vi "MA Scale Corrections.vi"(1 "RMC Calc Inputs":T1, 2 "Enable":bool=TRUE, 3 "MA Filter Size":i32=60, 8 "Reset":bool) -> (14 "RMC_Sm":dbl, 15 "RMC":dbl format="%.2f", 16 "Raw Weight":dbl format="%.2f", 17 "Corrected Weight":dbl format="%.2f", 18 "Wcomp":dbl, 19 "Wbouy":dbl)   [LabVIEW 2012]
uses:
  RMC Calc Inputs.ctl
  <vilib>/Analysis/baseanly.llb/Mean (DBL).vi
  <vilib>/Analysis/NI_AALBase.lvlib
panel:
  out "Smoothed Weight":dbl
  out "Count":dbl
  in  "Buoyancy Correction":T2={"Restriction"="3.75", "Bone Dry"=7.001999855041504, "Energie"=7, "Volume"=7.0, "IMC"=70.16566993034309, "Tamb"=70.16566993034309} {"Bone Dry" format="%.2f"}
  out "ColorW":bool
  in  "Period":u32
  in  "Data In":dbl[](array[numeric]) format="%.2f"
  out "Data Out":dbl[](array[numeric]) format="%.2f"
  in  "Compteur":u32
  in  "Bal_in":dbl=0.085 format="%.4f"
  out "Bal_out":dbl=0.085 format="%.4f"
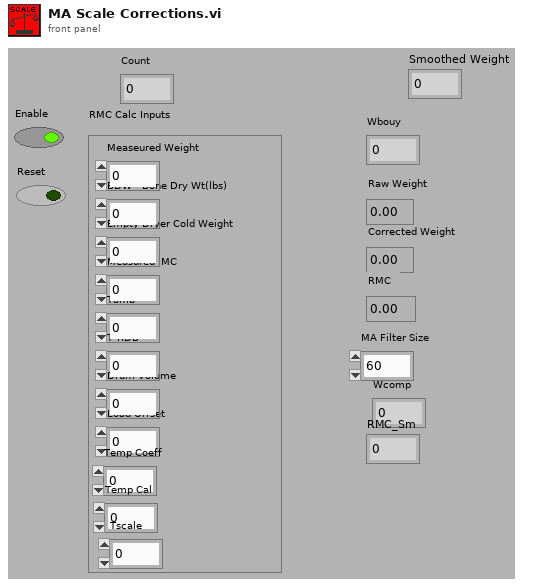
[diagram p1: front panel]
types:
  T1 = typedef "RMC Calc Inputs.ctl" = cluster{"Measeured Weight":dbl, "BDW - Bone Dry Wt(lbs)":dbl, "Empty Dryer Cold Weight":dbl, "Measured IMC":dbl, "Tamb":dbl, "T-RDB":dbl, "Drum Volume":dbl, "Load Offset":dbl, "Temp Coeff":dbl, "Temp Cal":dbl, "Tscale":dbl}
  T2 = cluster{"Restriction":string, "Bone Dry":dbl, "Energie":u8, "Volume":dbl, "IMC":dbl, "Tamb":dbl}
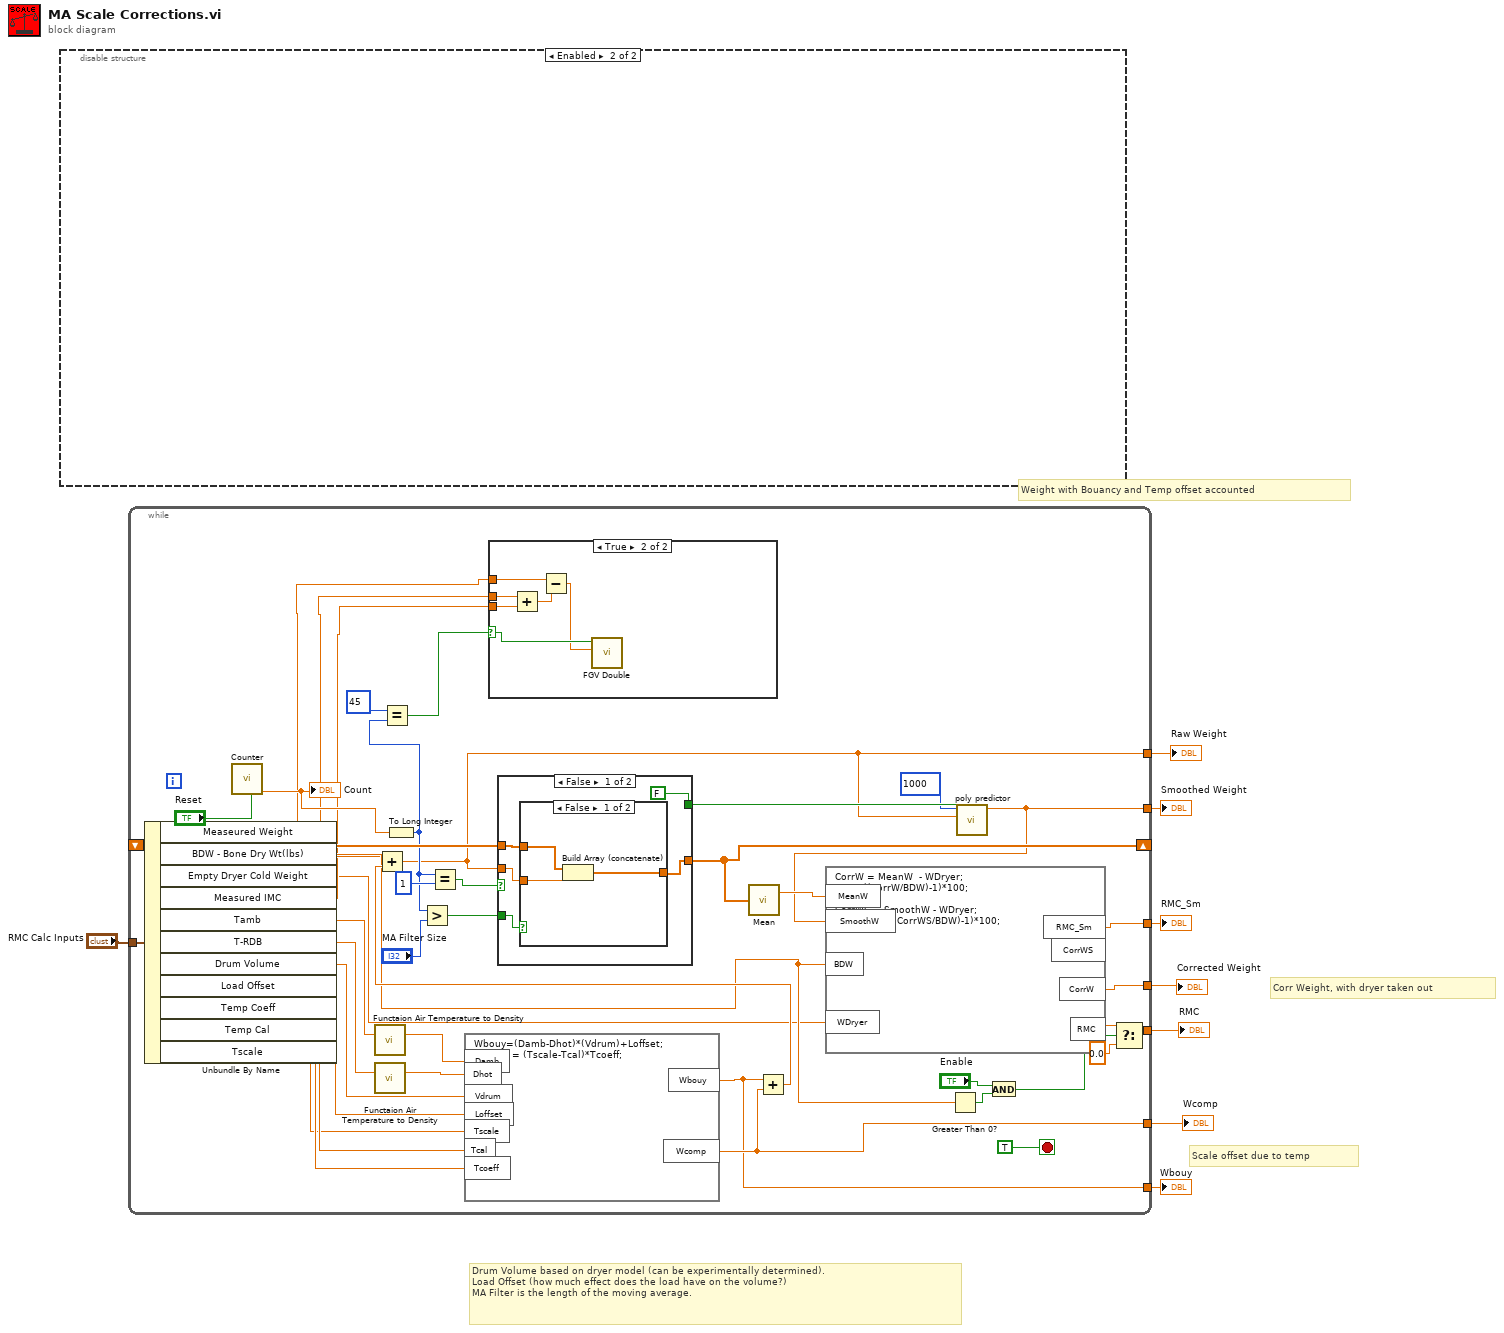
[diagram p0: block diagram]
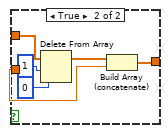
[diagram p3: hidden frame]
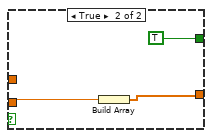
[diagram p4: hidden frame]
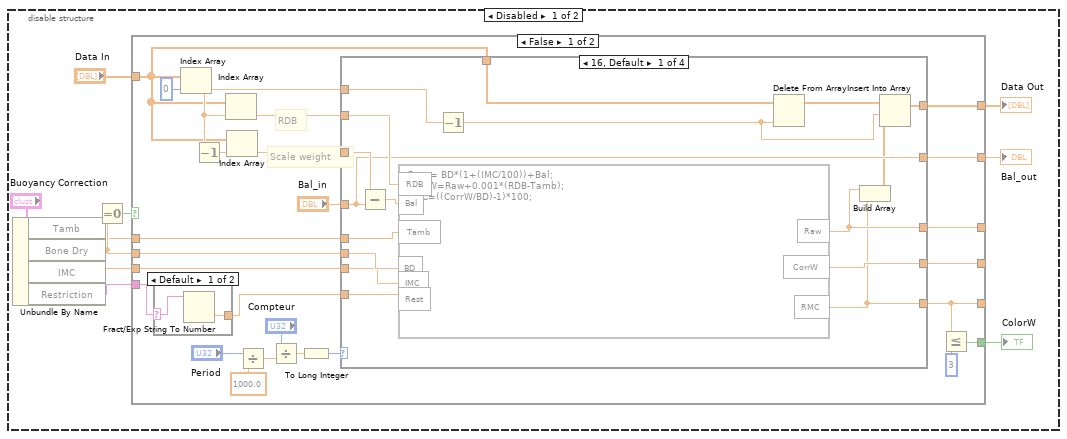
[diagram p5: hidden frame]
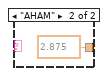
[diagram p6: hidden frame]
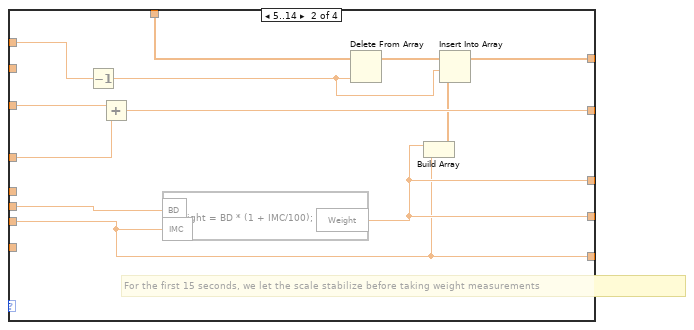
[diagram p7: hidden frame]
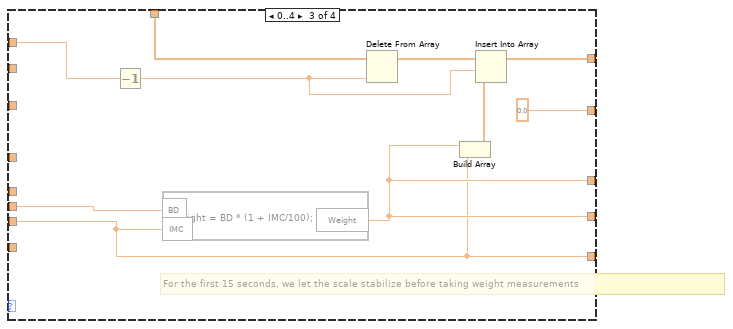
[diagram p8: hidden frame]
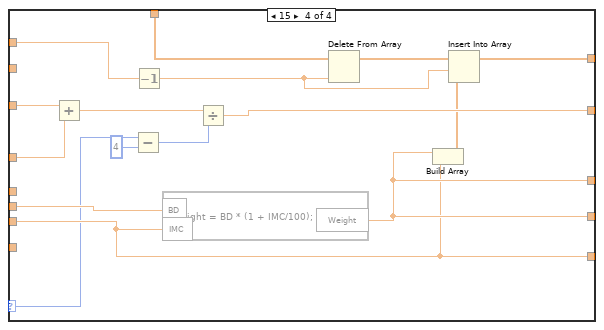
[diagram p9: hidden frame]
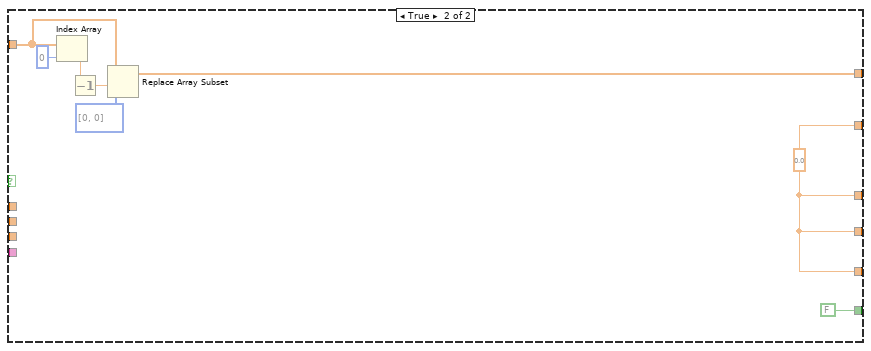
[diagram p10: hidden frame]
diagram:
  # "Corr Weight, with dryer taken out"
  # "Weight with Bouancy and Temp offset accounted"
  # "Scale offset due to temp"
  # "Drum Volume based on dryer model (can be experimentally determined).\nLoad Offset (how much effect does the load have on the volume?)\nMA Filter is the length of the moving average."
  n1 = disable-structure shown="Enabled" {
    frame Disabled {
      n2 = Unbundle By Name("Buoyancy Correction") -> ("Tamb"=w9:dbl, "Bone Dry"=w14:dbl, "IMC"=w13:dbl, "Restriction"=w12:string)
      n3 = Equal To 0?(x=w14) -> (x = 0?=w18:bool)
      n4 = case shown="False" w18 {
        tunnel: [w30 w103] -> _
        tunnel: [w29 w103] -> _
        tunnel: [w24 w103] -> _
        tunnel: "Data In" -> [w28 w107]
        tunnel: [w27 w104] -> w17
        tunnel: [w31 w103] -> w16
        tunnel: w14 -> [w26 _]
        tunnel: w13 -> [w25 _]
        tunnel: w12 -> [w21 _]
        tunnel: [w23 FALSE] -> w11
        tunnel: w9 -> [w19 _]
        frame False {
          # "RDB"
          # "Scale weight"
          n5 = case shown="Default" w21 {
            selector: w21 -> [w45 _]
            tunnel: [w44 2.875] -> w20
            frame Default {
              n6 = Fract/Exp String To Number(string=w45) -> (number=w44:dbl)  [unwired: 3 in, 1 out]
            }
            frame "AHAM" {
            }
          }
          n7 = Index Array(array=w28, index=0 ("Index")) -> (element=w41:dbl)
          n8 = Decrement(x=w41) -> (x-1=w42:dbl)
          n9 = Index Array(array=w28, index=w41) -> (element=w33:dbl)
          n10 = Index Array(array=w28, index=w42) -> (element=w34:dbl)
          n11 = Divide(x="Period", y=1000.0) -> (x/y=w38:dbl)
          n12 = Divide(x="Compteur", y=w38) -> (x/y=w36:dbl)
          n13 = To Long Integer(number=w36) -> (32bit integer=w37:i32)
          n14 = case shown="16, Default" w37 {
            selector: w37 -> [_ _ _ w89]
            tunnel: w34 -> [w58 w75 _ w101]
            tunnel: w33 -> [w60 _ _ _]
            tunnel: "Bal_in" -> [w57 w74 _ w100]
            tunnel: [w57 w73 0.0 ("Bal_in") w96] -> w31
            tunnel: w25 -> [w62 w66 w79 w91]
            tunnel: [w54 w66 w79 w91] -> w24
            tunnel: w26 -> [w63 w72 w85 w99]
            tunnel: w20 -> [w61 _ _ _]
            tunnel: [w55 w67 w80 w92] -> w30
            tunnel: [w56 w67 w80 w92] -> w29
            tunnel: w41 -> [w53 w69 w82 w95]
            tunnel: w28 -> [w52 w70 w83 w94]
            tunnel: [w50 w71 w84 w93] -> w27
            tunnel: w19 -> [w47 _ _ _]
            frame 16, Default {
              n15 = Subtract(x=w58, y=w57) -> (x-y=w59:dbl)
              n16 = formula code="Raw = BD*(1+(IMC/100))+Bal;\nCorrW=Raw+0.001*(RDB-Tamb);\nRMC=((CorrW/BD)-1)*100;"("Bal"=w59, "BD"=w63, "IMC"=w62, "Rest"=w61, "RDB"=w60, "Tamb"=w47) -> ("Raw"=w55:dbl, "CorrW"=w56:dbl, "RMC"=w54:dbl)
              n17 = Decrement(x=w53) -> (x-1=w48:dbl)
              n18 = Delete From Array(array=w52, index=w48) -> (array with subset deleted=w49:dbl[])  [unwired: 1 in, 1 out]
              n19 = Build Array(w55, w54) -> (w51:dbl[])
              n20 = Insert Into Array(array=w49, index=w48, new element=w51) -> (w50:dbl[])
            }
            frame 5..14 {
              # "For the first 15 seconds, we let the scale stabilize before taking weight measurements"
              n21 = Decrement(x=w69) -> (x-1=w64:dbl)
              n22 = Add(x=w75, y=w74) -> (x+y=w73:dbl)
              n23 = formula code="Weight = BD * (1 + IMC/100);"("BD"=w72, "IMC"=w66) -> ("Weight"=w67:dbl)
              n24 = Delete From Array(array=w70, index=w64) -> (array with subset deleted=w65:dbl[])  [unwired: 1 in, 1 out]
              n25 = Build Array(w67, w66) -> (w68:dbl[])
              n26 = Insert Into Array(array=w65, index=w64, new element=w68) -> (w71:dbl[])
            }
            frame 0..4 {
              # "For the first 15 seconds, we let the scale stabilize before taking weight measurements"
              n27 = Decrement(x=w82) -> (x-1=w76:dbl)
              n28 = formula code="Weight = BD * (1 + IMC/100);"("BD"=w85, "IMC"=w79) -> ("Weight"=w80:dbl)
              n29 = Delete From Array(array=w83, index=w76) -> (array with subset deleted=w77:dbl[])  [unwired: 1 in, 1 out]
              n30 = Build Array(w80, w79) -> (w81:dbl[])
              n31 = Insert Into Array(array=w77, index=w76, new element=w81) -> (w84:dbl[])
            }
            frame 15 {
              n32 = Add(x=w101, y=w100) -> (x+y=w98:dbl)
              n33 = Subtract(x=w89, y=4) -> (x-y=w97:i32)
              n34 = Decrement(x=w95) -> (x-1=w86:dbl)
              n35 = formula code="Weight = BD * (1 + IMC/100);"("BD"=w99, "IMC"=w91) -> ("Weight"=w92:dbl)
              n36 = Divide(x=w98, y=w97) -> (x/y=w96:dbl)
              n37 = Delete From Array(array=w94, index=w86) -> (array with subset deleted=w87:dbl[])  [unwired: 1 in, 1 out]
              n38 = Build Array(w92, w91) -> (w90:dbl[])
              n39 = Insert Into Array(array=w87, index=w86, new element=w90) -> (w93:dbl[])
            }
          }
          n40 = Less Or Equal?(x=w24, y=i8 3) -> (x <= y?=w23:bool)
        }
        frame True {
          w103 = 0.0
          n41 = Index Array(array=w107, index=0 ("Index")) -> (element=w108:dbl)
          n42 = Decrement(x=w108) -> (x-1=w106:dbl)
          n43 = Replace Array Subset(array=w107, new element=i32[] [0, 0] ("Array Constant"), index=w106) -> (w104:dbl[])
        }
      }
      "Data Out" <- w17
      "Bal_out" <- w16
      "ColorW" <- w11
    }
    frame Enabled {
    }
  }
  n44 = while {
    tunnel: "RMC Calc Inputs" -> [w150]
    shift-right: [w148] -> _
    shift-left: _ -> [w149]
    tunnel: [w130] -> w8
    tunnel: [w114] -> w7
    tunnel: [w146] -> w6
    tunnel: [w128] -> w4
    tunnel: [w122] -> w3
    tunnel: [w119] -> w2
    tunnel: [w117] -> w1
    stop <- TRUE stop-if-true
    n45 = Unbundle By Name(w150) -> ("Measeured Weight"=w112:dbl, "BDW - Bone Dry Wt(lbs)"=w124:dbl, "Empty Dryer Cold Weight"=w110:dbl, "Measured IMC"=w111:dbl, "Tamb"=w141:dbl, "T-RDB"=w140:dbl, "Drum Volume"=w138:dbl, "Load Offset"=w139:dbl, "Temp Coeff"=w135:dbl, "Temp Cal"=w134:dbl, "Tscale"=w132:dbl)
    n46 = call "Counter.vi"("Reset"="Reset") -> ("Count"=w123:dbl)  [unwired: 10 in]
    "Count" <- w123
    n47 = call "Functaion Air Temperature to Density.vi"("Temp(F)"=w141) -> ("Density (lb/ft3)"=w137:dbl)  [unwired: 14 in]
    n48 = call "Functaion Air Temperature to Density.vi"("Temp(F)"=w140) -> ("Density (lb/ft3)"=w136:dbl)  [unwired: 14 in]
    n49 = To Long Integer(number=w123) -> (32bit integer=w115:i32)
    n50 = Equal?(x=45 ("y"), y=w115) -> (x = y?=w113:bool)
    n51 = Greater?(x=w115, y="MA Filter Size") -> (0:w142:bool)
    n52 = Equal?(x=w115, y=1) -> (x = y?=w145:bool)
    n53 = formula code="Wbouy=(Damb-Dhot)*(Vdrum)+Loffset;\nWcomp = (Tscale-Tcal)*Tcoeff;"("Damb"=w137, "Dhot"=w136, "Vdrum"=w138, "Loffset"=w139, "Tscale"=w132, "Tcal"=w134, "Tcoeff"=w135) -> ("Wbouy"=w122:dbl, "Wcomp"=w128:dbl)
    n54 = case shown="True" w113 {
      selector: w113 -> [_ w157]
      tunnel: w112 -> [_ w156]
      tunnel: w111 -> [_ w155]
      tunnel: w110 -> [_ w154]
      frame False {
      }
      frame True {
        n55 = Add(x=w154, y=w155) -> (x+y=w153:dbl)
        n56 = Subtract(x=w156, y=w153) -> (x-y=w152:dbl)
        n57 = call "FGV Double.vi"("Value In"=w152, "Set?"=w157) -> ()  [unwired: 9 in, 1 out]
      }
    }
    n58 = Add(x=w122, y=w128) -> (x+y=w133:dbl)
    n59 = Add(x=w112, y=w133) -> (x+y=w114:dbl)
    n60 = case shown="False" w145 {
      tunnel: w114 -> [w162 w174]
      tunnel: w149 -> [w161 _]
      tunnel: [w160 w173] -> w148
      tunnel: w142 -> [w159 _]
      tunnel: [FALSE TRUE] -> w120
      frame False {
        n61 = case shown="False" w159 {
          tunnel: [w165 w166] -> w160
          tunnel: w162 -> [w164 w167]
          tunnel: w161 -> [w163 w171]
          frame False {
            n62 = Build Array (concatenate)(w163, w164) -> (w165:dbl[])
          }
          frame True {
            n63 = Delete From Array(array=w171, length=1, index=0) -> (array with subset deleted=w168:dbl[])  [unwired: 1 out]
            n64 = Build Array (concatenate)(w168, w167) -> (w166:dbl[])
          }
        }
      }
      frame True {
        n65 = Build Array(w174) -> (w173:dbl[])
      }
    }
    n66 = call-poly <vilib>:"Mean.vi"("X"=w148) -> ("mean"=w147:dbl)  [unwired: 1 out]
    n67 = Greater Than 0?(x=w124) -> (x > 0?=w126:bool)
    n68 = call "poly predictor.vi"("Initialize"=w120, "Weight"=w114, "Number of Values to Smooth"=1000) -> ("Smoothed Value"=w119:dbl)  [unwired: 8 in]
    n69 = formula code="CorrW = MeanW  - WDryer;\nRMC=((CorrW/BDW)-1)*100;\n\nCorrWS = SmoothW - WDryer;\nRMC_Sm = ((CorrWS/BDW)-1)*100;"("BDW"=w124, "MeanW"=w147, "WDryer"=w110, "SmoothW"=w119) -> ("CorrW"=w146:dbl, "RMC"=w131:dbl, "RMC_Sm"=w117:dbl)  [unwired: 1 out]
    n70 = And(x="Enable", y=w126) -> (x .and. y?=w125:bool)
    n71 = Select(t=w131, s=w125, f=0.0) -> (s? t:f=w130:dbl)
  }
  "RMC" <- w8
  "Corrected Weight" <- w6
  "Raw Weight" <- w7
  "Wcomp" <- w4
  "Wbouy" <- w3
  "Smoothed Weight" <- w2
  "RMC_Sm" <- w1
